vi "Log String Message.vi"(8 "Error In":errorcluster, 10 "Message":string, 11 "UILogger In":refnum<class "UILogger.lvclass">) -> (0 "Error Out":errorcluster, 3 "UILogger Out":refnum<class "UILogger.lvclass">)   [LabVIEW 2019, in "UILogger.lvclass"]
uses:
  UILogger.lvclass
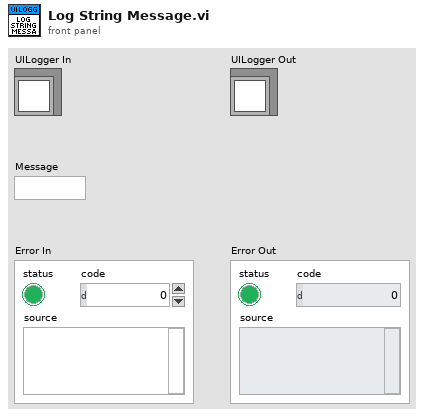
[diagram p1: front panel]
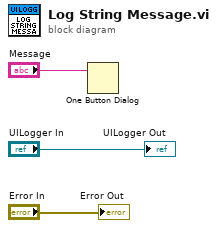
[diagram p0: block diagram]
diagram:
  n1 = One Button Dialog(message="Message") -> ()  [unwired: 1 in, 1 out]
  "Error Out" <- "Error In"
  "UILogger Out" <- "UILogger In"
